vi "Image translate (from file).vi"(0 "Image file path":path=path "C:/Users/Paul Nathan/Desktop/Turntable test 3/Datum_Turntable_2.jpg", 1 "Translated image file path":path=path "C:/Users/Paul Nathan/Desktop/Turntable test 3/Datum_Turntable_2_X.jpg", 2 "Tx (pixels)":dbl, 3 "Ty (pixels)":dbl, 4 "Quality":u32=750 max=1000, 5 "Error in":errorcluster) -> (19 "Error Out":errorcluster)   [LabVIEW 2015]
panel:
  out "Image out":T1(plugin-control)
  # "PN 18/03/2016"
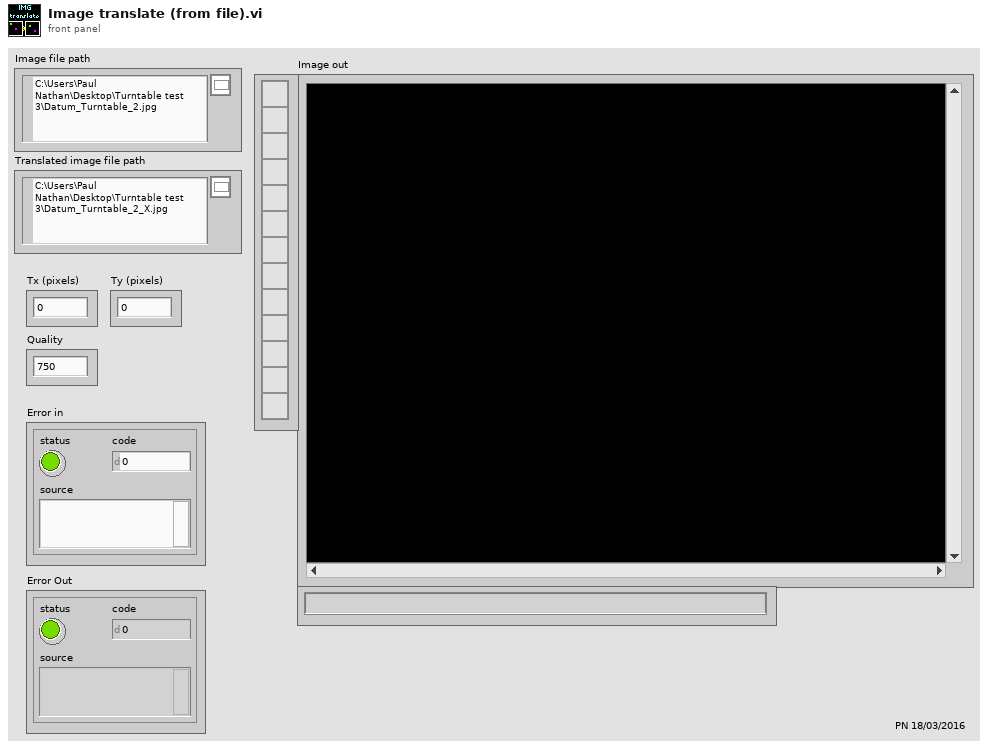
[diagram p1: front panel]
types:
  T1 = typedef "IMAQ Image.ctl" = refnum<image>
  T2 = typedef "Image Type" = u32
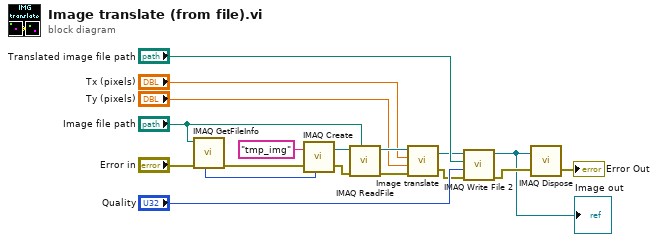
[diagram p0: block diagram]
diagram:
  n1 = call "IMAQ GetFileInfo"("error in (no error)"="Error in", "File Path"="Image file path") -> ("error out"=w15:errorcluster, "Image Type"=w14:T2)  [unwired: 3 in, 5 out]
  n2 = call "IMAQ Create"("Image Name"="tmp_img", "Image Type"=w14, "error in (no error)"=w15) -> ("New Image"=w17:T1, "error out"=w16:errorcluster)  [unwired: 2 in]
  n3 = call "IMAQ ReadFile"("File Path"="Image file path", "error in (no error)"=w16, "Image"=w17) -> ("error out"=w6:errorcluster, "Image Out"=w3:T1)  [unwired: 4 in, 3 out]
  n4 = call "Image translate.vi"("Error in"=w6, "Ty (pix)"="Ty (pixels)", "Tx (pix)"="Tx (pixels)", "Image in"=w3) -> ("Error Out"=w5:errorcluster, "Image Out"=w4:T1)
  n5 = call-poly "IMAQ Write File 2"("error in (no error)"=w5, "Image Quality"="Quality", "File Path"="Translated image file path", "Image"=w4) -> ("error out"=w13:errorcluster, "Image Out (duplicate)"=w9:T1)  [unwired: 6 in]
  "Image out" <- w9
  n6 = call "IMAQ Dispose"("Image"=w9, "error in (no error)"=w13) -> ("error out"=→"Error Out":errorcluster)  [unwired: 4 in]
